vi "CSM - Module Turns Invalid.vi"(3 "CSM Name":string) -> (1 "Turn Invalid(Exit)?":bool)   [LabVIEW 2020, in "Communicable State Machine.lvlib"]
doc: "Check if CSM module is not valid any more. This is usually used in sub-loops with a CSM for acting as a holistic module. It's used for exit condition of the sub-loops.\n\n<b>Inputs:</b>\n - <b>CSM Name</b>: Host Module Name\n\n<b>Outputs:</b>\n - <b>Turn Invalid(Exit)?</b>: CSM Module turns invalid"
uses:
  Communicable State Machine.lvlib
  global-CSMQ FGV Change Flag.vi
  _CSMOFGV.vi
  Priority Queue.lvclass
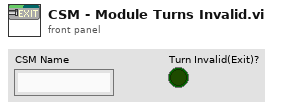
[diagram p1: front panel]
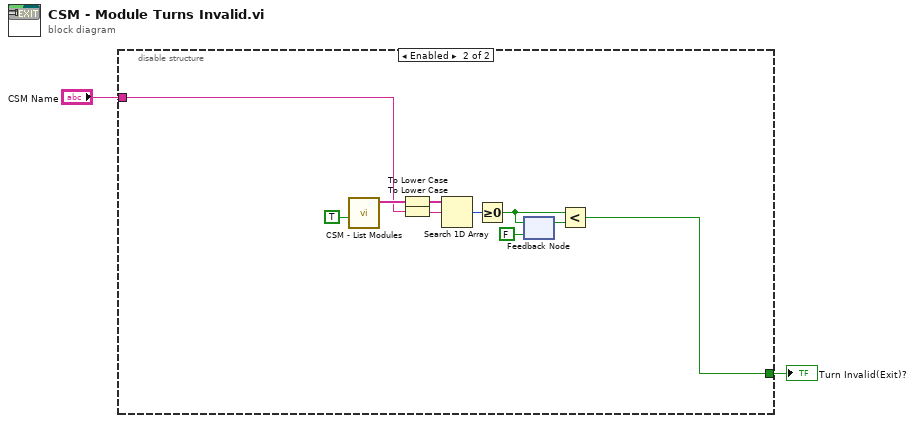
[diagram p0: block diagram]
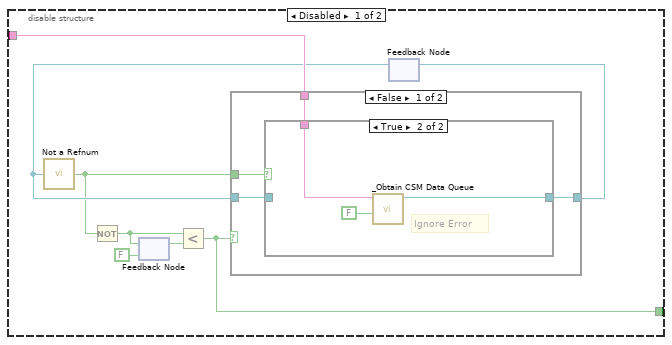
[diagram p2: hidden frame]
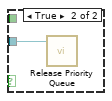
[diagram p4: hidden frame]
diagram:
  n1 = disable-structure shown="Enabled" {
    disable-tunnel: "CSM Name" -> [w10 w27]
    disable-tunnel: [w3 w20] -> w1
    frame Disabled {
      n2 = feedback #1(FALSE) -> (w7:bool)
      n3 = feedback #2() -> (w9:refnum<class "Priority Queue.lvclass">)  [unwired: 1 in]
      n4 = call "Not a Refnum.vi"("Priority Queue.lvclass"=w9) -> ("NaN/Path/Refnum?"=w4:bool)  [unwired: 4 in]
      n5 = Not(x=w4) -> (.not. x?=w8:bool)
      n6 = feedback-in #1(w8) -> ()
      n7 = Less?(x=w8, y=w7) -> (x < y?=w3:bool)
      n8 = case shown="False" w3 {
        tunnel: w10 -> [w14 _]
        tunnel: w9 -> [w13 w19]
        tunnel: [w12 _] -> w5
        tunnel: w4 -> [w11 _]
        frame False {
          n9 = case shown="True" w11 {
            tunnel: w14 -> [_ w18]
            tunnel: [w15 w16] -> w12
            tunnel: w13 -> [w15 _]
            frame False {
            }
            frame True {
              # "Ignore Error"
              n10 = call "_Obtain CSM Data Queue.vi"("create if not found? (T)"=FALSE, "Name"=w18) -> ("Priority Queue"=w16:refnum<class "Priority Queue.lvclass">)  [unwired: 7 in, 2 out]
            }
          }
        }
        frame True {
          n11 = call "Release Priority Queue.vi"("Priority Queue"=w19) -> ()  [unwired: 10 in, 1 out]
        }
      }
      n12 = feedback-in #2(w5) -> ()
    }
    frame Enabled {
      n13 = call "CSM - List Modules.vi"("All?"=TRUE) -> ("Module Names"=w28:string[])  [unwired: 9 in, 1 out]
      n14 = To Lower Case(string=w28) -> (all lower case string=w26:string[])
      n15 = To Lower Case(string=w27) -> (all lower case string=w25:string)
      n16 = Search 1D Array(1D array=w26, element=w25) -> (index of element=w21:i32)  [unwired: 1 in]
      n17 = Greater Or Equal To 0?(x=w21) -> (x >= 0?=w24:bool)
      n18 = feedback #3(FALSE) -> (w23:bool)
      n19 = feedback-in #3(w24) -> ()
      n20 = Less?(x=w24, y=w23) -> (x < y?=w20:bool)
    }
  }
  "Turn Invalid(Exit)?" <- w1
